vi "Simulated Database.vi"(11 "Function":T2) -> ()   [LabVIEW 2011]
uses:
  DataType/Simulated Database_Function.ctl
  DataType/Simulated Database_Record.ctl
panel:
  out "Record":T1 {"Balance" format="%9.2f"; "Account Number" format="%0#5_5g"}
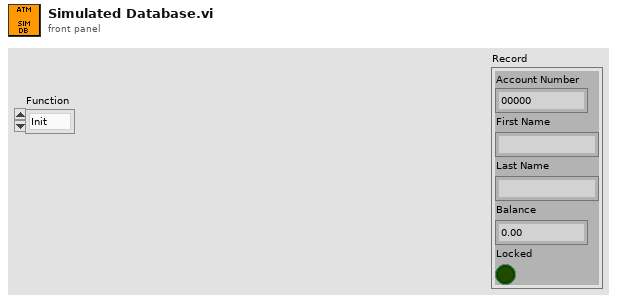
[diagram p1: front panel]
types:
  T1 = typedef "Simulated Database_Record.ctl" = cluster{"Account Number":dbl, "First Name":string, "Last Name":string, "Balance":dbl, "Locked":bool}
  T2 = typedef "Simulated Database_Function.ctl" = enum16{"Init", "Search account and lock record", "Modify balance", "Access record", "Commit record", "Unlock record"}
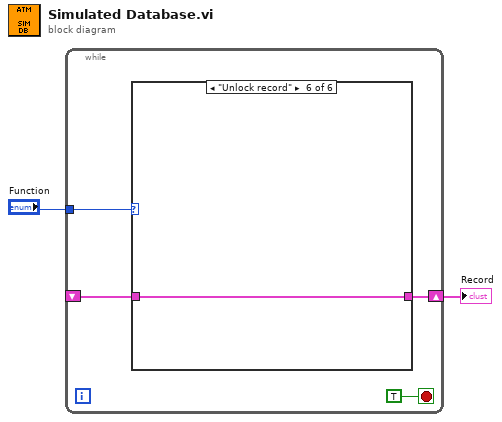
[diagram p0: block diagram]
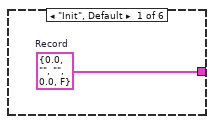
[diagram p2: hidden frame]
diagram:
  n1 = while {
    tunnel: "Function" -> [w5]
    shift-right: [w4] -> w1
    shift-left: _ -> [w3]
    stop <- TRUE stop-if-true
    n2 = case shown="\"Unlock record\"" w5 {
      tunnel: [w7 w8 w9 w10 w11 w12] -> w4
      tunnel: w3 -> [_ w8 w9 w10 w11 w12]
      frame "Init", Default {
        w7 = T1 {"Account Number"=0.0, "First Name"="", "Last Name"="", "Balance"=0.0, "Locked"=FALSE}  # Record
      }
      frame "Search account and lock record" {
      }
      frame "Modify balance" {
      }
      frame "Access record" {
      }
      frame "Commit record" {
      }
      frame "Unlock record" {
      }
    }
  }
  "Record" <- w1
